vi "Create Tree.vi"(7 "Parent ID (empty)":string, 8 "Error In":errorcluster, 10 "Name":string, 11 "Tree Manager":T1) -> (0 "Error Out":errorcluster, 3 "Tree Manager":T1, 5 "Unique ID":string)   [LabVIEW 2020, in "NI_VIAnCFGDataStructure.lvlib" / "Tree.lvclass"]
doc: "Create a new Tree in the Tree Manager and assign to it a Unique ID. Use this Unique ID to interact with this tree.\n\nYou can provide the optional Parent ID input if you want to create the Child Tree directly under already existing Parent.\n\n<b>WARNING</b> The name Attr is reserved by the Tree API. Do not use that name for your Trees. Flattening to XML requires the Tree Names to contain no white spaces. All white spaces will be replaced with underscore characters when flattening."
uses:
  <vilib>/addons/analyzer/VIAnCFGDataStructure/Tree Manager/Tree.lvclass
  <vilib>/addons/analyzer/VIAnCFGDataStructure/Tree Manager/Typedefs/Session Handle.ctl
  <vilib>/addons/analyzer/VIAnCFGDataStructure/Tree Manager/Tree.lvclass/Tree.ctl
  <vilib>/Utility/error.llb/Error Cluster From Error Code.vi
  <vilib>/ErrorRing/Error Ring.xnode
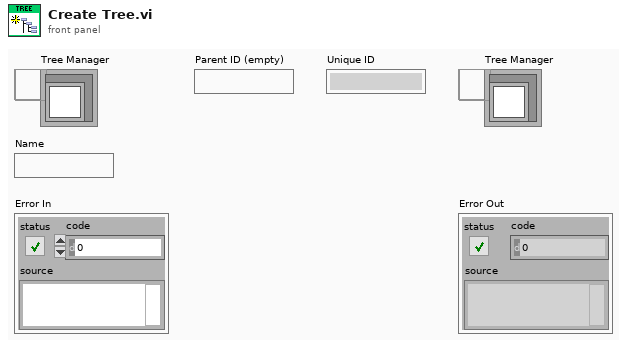
[diagram p1: front panel]
types:
  T1 = typedef "NI_VIAnCFGDataStructure.lvlib/Tree.lvclass/Session Handle.ctl" = refnum<data-value>
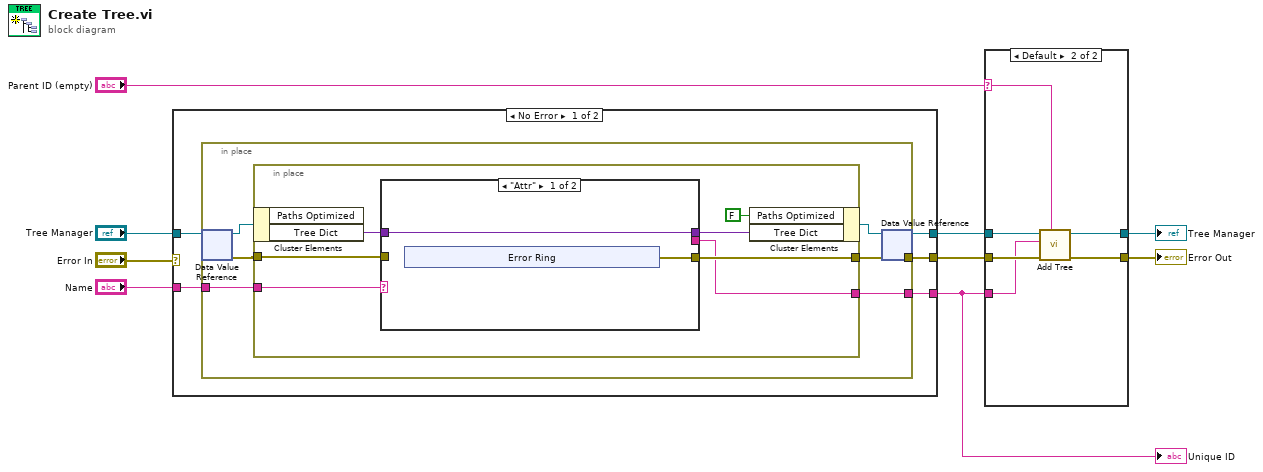
[diagram p0: block diagram]
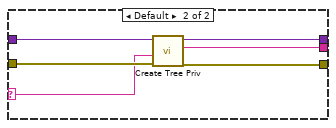
[diagram p3: hidden frame]
diagram:
  n1 = case shown="No Error" "Error In" {
    selector: "Error In" -> [_ w41]
    tunnel: "Tree Manager" -> [w14 w42]
    tunnel: [w13 w42] -> w7
    tunnel: [w12 w41] -> w8
    tunnel: "Name" -> [w11 _]
    tunnel: [w10 _] -> w5
    frame No Error {
      n2 = in-place {
        in-place-border: [w19] -> w12
        in-place-border: w11 -> [w17]
        in-place-border: [w16] -> w10
        n3 = in-place-dvr #1(w14) -> (w20:refnum<class "Tree.lvclass">, w15:errorcluster)
        n4 = in-place {
          in-place-border: [w24] -> w19
          in-place-border: w15 -> [w25]
          in-place-border: w17 -> [w22]
          in-place-border: [w23] -> w16
          n5 = in-place-cluster #2(w20) -> ("Tree Dict"=w27:variant)  [unwired: 1 out]
          n6 = case shown="\"Attr\"" w22 {
            selector: w22 -> [_ w35]
            tunnel: w27 -> [w29 w40]
            tunnel: [w29 w39] -> w26
            tunnel: w25 -> [_ w38]
            tunnel: [w28 w37] -> w24
            tunnel: [_ w36] -> w23
            frame "Attr" {
              n7 = xnode "Error Ring"() -> ("error out"=w28:errorcluster)
            }
            frame Default {
              n8 = call <vilib>:"Create Tree Priv.vi"("Error In"=w38, "Name"=w35, "Tree Dictionary In"=w40) -> ("Error Out"=w37:errorcluster, "Unique ID"=w36:string, "Tree Dictionary Out"=w39:variant)  [unwired: 6 in]
            }
          }
          n9 = in-place-cluster #2("Paths Optimized"=FALSE, "Tree Dict"=w26) -> (w18:refnum<class "Tree.lvclass">)
        }
        n10 = in-place-dvr #1(w18) -> (w13:T1)  [unwired: 1 out]
      }
    }
    frame Error {
    }
  }
  "Unique ID" <- w5
  n11 = case shown="Default" "Parent ID (empty)" {
    selector: "Parent ID (empty)" -> [_ w46]
    tunnel: w8 -> [w43 w50]
    tunnel: [w43 w49] -> w1
    tunnel: w7 -> [w44 w48]
    tunnel: [w44 w47] -> w2
    tunnel: w5 -> [_ w45]
    frame "" {
    }
    frame Default {
      n12 = call <vilib>:"Add Tree.vi"("Parent ID"=w46, "Error In"=w50, "Child ID"=w45, "Tree Manager"=w48) -> ("Error Out"=w49:errorcluster, "Tree Manager"=w47:T1)  [unwired: 6 in]
    }
  }
  "Tree Manager" <- w2
  "Error Out" <- w1
